vi "Buffer Classes Test.vi"() -> ()   [LabVIEW 2012]
uses:
  Engine/Classes/Waveforms/Buffer/Waveform Buffer/Waveform Buffer.lvclass
  Engine/Classes/Waveforms/Buffer/DBL Waveform Buffer/DBL Waveform Buffer.lvclass
  Engine/Classes/Waveforms/Buffer/Waveform Buffer/Buffer Data Type.ctl
  Engine/Classes/Waveforms/Buffer/Waveform Buffer/Time Range.ctl
  Engine/Classes/Waveforms/Buffer/Waveform Buffer/Data Point.ctl
  Engine/Classes/Waveforms/Buffer/Waveform Buffer/Wfm Segment.ctl
panel:
  out "DBL Buffer":refnum<class "DBL Waveform Buffer.lvclass">
  out "Cluster":T1={"Data"=[3000.0, 3001.0, 3002.0, 3003.0, 3004.0, 3005.0, 3006.0, 3007.0, 3008.0, 3009.0, 3010.0, 3011.0], "Segment Info"={"New Segment"=TRUE, "Wfm time"=timestamp(3449251614.0738325 s since 1904-01-01)}, "dt"=0.001}
  out "current time":timestamp=timestamp(3449251579.04933 s since 1904-01-01)
  out "Data":cluster{"Data":dbl[]}[](array[cluster])=[{"Data"=[3000.0, 3001.0, 3002.0, 3003.0, 3004.0, 3005.0, 3006.0, 3007.0, 3008.0, 3009.0, 3010.0, 3011.0]}]
  out "Wfm Segments":T2[](array[typedef])=[{"ID"=3, "Total samples"=12, "Start"={"Index"=0, "Wfm time"=timestamp(3449251614.0738325 s since 1904-01-01), "Receive time"=timestamp(3449251614.0738325 s since 1904-01-01)}, "Finish"={"Index"=11, "Wfm time"=timestamp(3449251614.0858326 s since 1904-01-01), "Receive time"=timestamp(3449251614.0858326 s since 1904-01-01)}}]
  in  "Read Wfms":bool
  in  "Time Range":T4={"Use Receive Time"=FALSE, "Start Time"=timestamp(3417715391.753 s since 1904-01-01), "Stop time"=timestamp(3480787391.753 s since 1904-01-01)}
  out "Waveform Buffer":refnum<class "Waveform Buffer.lvclass">
  in  "Send Wfm":bool
  in  "Wfm":T5={"New Segment"=TRUE, "dt"=0.001, "Wfm size"=12}
  in  "stop":bool
  in  "Buffer Duration":dbl=2.0
  in  "Buffer Data Type":T6
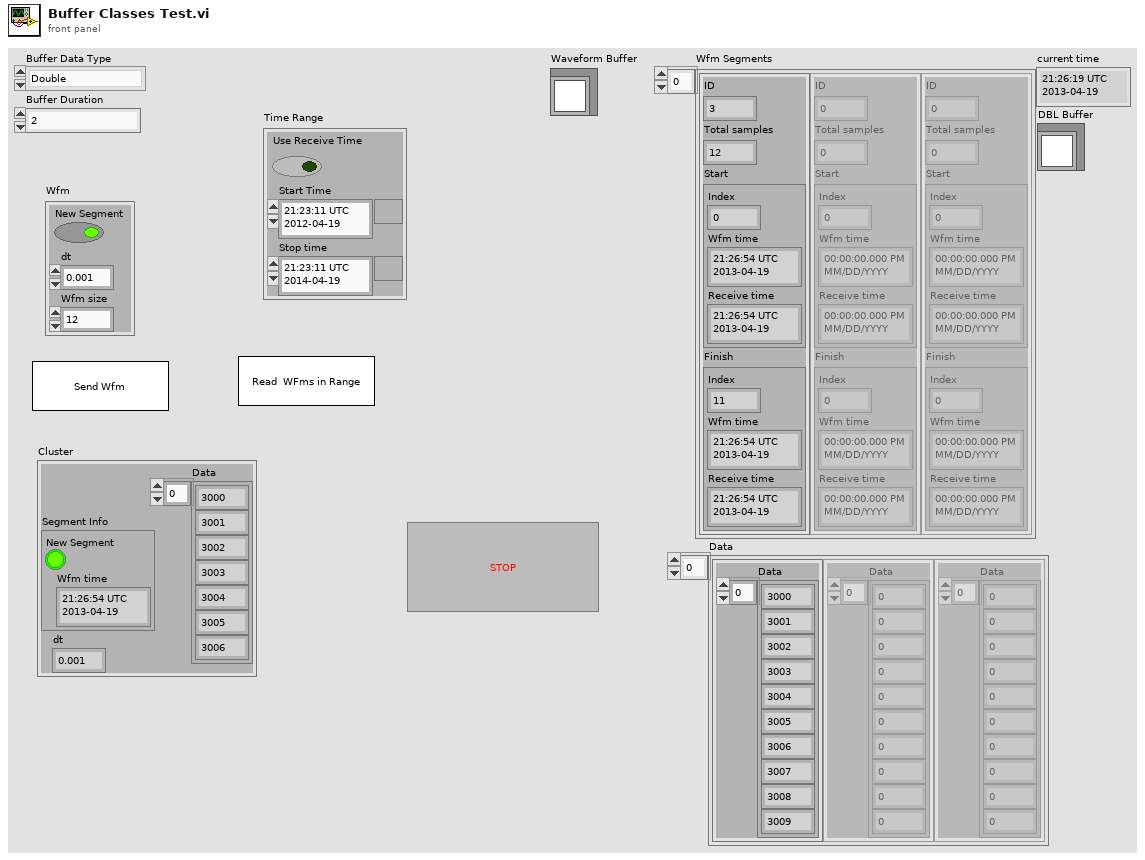
[diagram p1: front panel]
types:
  T1 = cluster{"Data":dbl[], "Segment Info":cluster{"New Segment":bool, "Wfm time":timestamp}, "dt":dbl}
  T2 = typedef "Waveform Data Logger Engine.lvlib/Waveform Buffer.lvclass/Wfm Segment.ctl" = cluster{"ID":u64, "Total samples":i32, "Start":T3, "Finish":T3}
  T3 = typedef "Waveform Data Logger Engine.lvlib/Waveform Buffer.lvclass/Data Point.ctl" = cluster{"Index":i32, "Wfm time":timestamp, "Receive time":timestamp}
  T4 = typedef "Waveform Data Logger Engine.lvlib/Waveform Buffer.lvclass/Time Range.ctl" = cluster{"Use Receive Time":bool, "Start Time":timestamp, "Stop time":timestamp}
  T5 = cluster{"New Segment":bool, "dt":dbl, "Wfm size":i32}
  T6 = typedef "Waveform Data Logger Engine.lvlib/Waveform Buffer.lvclass/Buffer Data Type.ctl" = enum16{"Double", "ComplexDouble"}
  T7 = cluster{"New Segment":bool, "Wfm time":timestamp, "Receive time":timestamp}
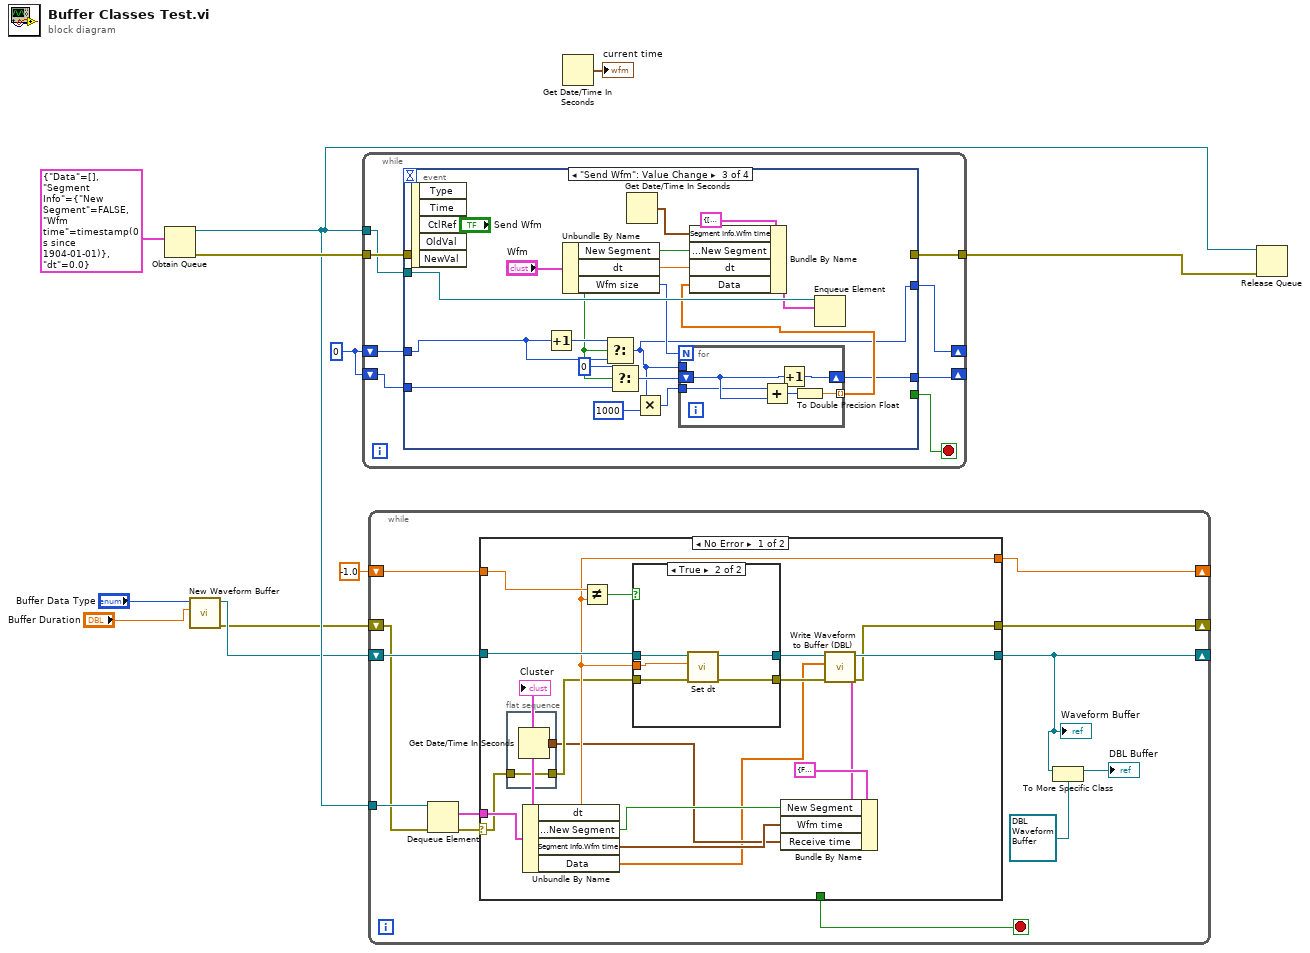
[diagram p0: block diagram]
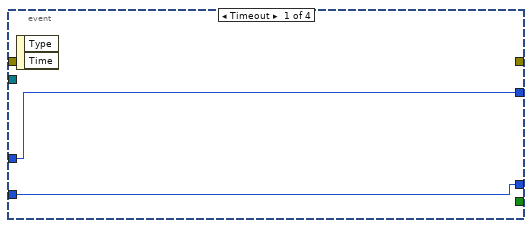
[diagram p2: hidden frame]
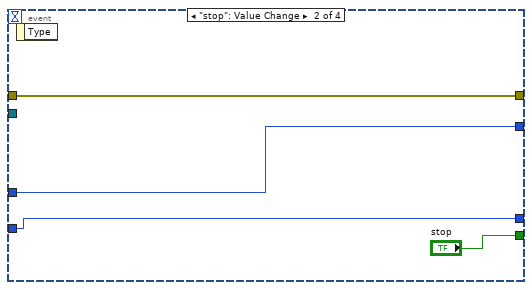
[diagram p3: hidden frame]
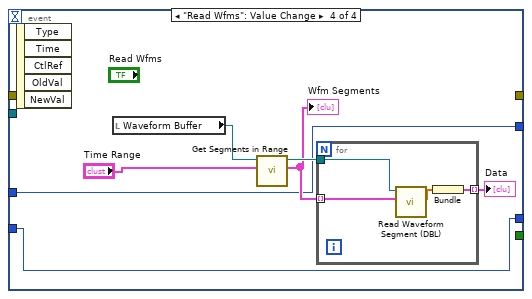
[diagram p4: hidden frame]
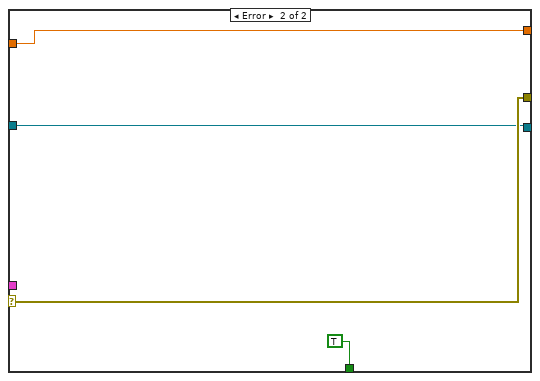
[diagram p6: hidden frame]
diagram:
  w5 = 0
  n1 = Obtain Queue(element data type=T1 {"Data"=[], "Segment Info"={"New Segment"=FALSE, "Wfm time"=timestamp(0 s since 1904-01-01)}, "dt"=0.0}) -> (queue out=w7:refnum<queue>, error out=w9:errorcluster)  [unwired: 4 in, 1 out]
  n2 = call "New Waveform Buffer.vi"("Buffer Duration"="Buffer Duration", "Buffer Data Type"="Buffer Data Type") -> ("error out"=w3:errorcluster, "Waveform Buffer out"=w4:refnum<class "Waveform Buffer.lvclass">)  [unwired: 8 in]
  n3 = while {
    tunnel: w7 -> [w14]
    tunnel: w9 -> [w17]
    tunnel: [w18] -> w8
    shift-right: [w16] -> _
    shift-left: w5 -> [w15]
    shift-right: [w12] -> _
    shift-left: w5 -> [w13]
    stop <- w19 stop-if-true
    n4 = event shown="[2] \"Send Wfm\": Value Change" {
      selector: _ -> [_ _ _ _]
      dyn-events: _ -> [_ _ _ _]
      timeout: _ -> [_ _ _ _]
      tunnel: [_ "stop" _ _] -> w19
      tunnel: [_ w24 _ _] -> w18
      tunnel: w17 -> [_ w24 _ _]
      tunnel: [w21 w23 w29 w50] -> w16
      tunnel: w15 -> [w21 w23 w41 w50]
      tunnel: w14 -> [_ _ w40 _]
      tunnel: w13 -> [w20 w22 w34 w49]
      tunnel: [w20 w22 w30 w49] -> w12
      event Timeout {
        n5 = event-data() -> ()  [unwired: 1 in, 2 out]
      }
      event "stop": Value Change {
        n6 = event-data() -> ()  [unwired: 1 in, 1 out]
      }
      event "Send Wfm": Value Change {
        n7 = event-data() -> ()  [unwired: 1 in, 5 out]
        n8 = Increment(x=w41) -> (x+1=w42:i32)
        n9 = Unbundle By Name("Wfm") -> ("New Segment"=w36:bool, "dt"=w38:dbl, "Wfm size"=w37:i32)
        n10 = Select(t=w42, s=w36, f=w41) -> (s? t:f=w29:i32)
        n11 = Select(t=0, s=w36, f=w34) -> (s? t:f=w33:i32)
        n12 = Get Date/Time In Seconds() -> (seconds since 1Jan1904=w26:timestamp)
        n13 = Multiply(x=w29, y=1000) -> (x*y=w27:i32)
        n14 = for {
          N: w37 -> [_]
          shift-right: [w46] -> w30
          shift-left: w33 -> [w45]
          tunnel: w29 -> [_]
          tunnel: [w47] -> w32 mode=indexing
          tunnel: w27 -> [w44]
          n15 = Add(x=w44, y=w45) -> (x+y=w48:i32)
          n16 = Increment(x=w45) -> (x+1=w46:i32)
          n17 = To Double Precision Float(number=w48) -> (double precision float=w47:dbl)
        }
        n18 = Bundle By Name(cluster=T1 {"Data"=[], "Segment Info"={"New Segment"=FALSE, "Wfm time"=timestamp(0 s since 1904-01-01)}, "dt"=0.0}, "Segment Info.Wfm time"=w26, "Segment Info.New Segment"=w36, "dt"=w38, "Data"=w32) -> (w31:T1)
        n19 = Enqueue Element(queue=w40, element=w31) -> ()  [unwired: 2 in, 3 out]
      }
      event "Read Wfms": Value Change {
        n20 = event-data() -> ()  [unwired: 1 in, 5 out]
        n21 = local read "Waveform Buffer"() -> (w55:refnum<class "Waveform Buffer.lvclass">)
        n22 = call "Get Segments in Range.vi"("Time Range"="Time Range", "Waveform Buffer in"=w55) -> ("Wfm Segments"=w52:T2[], "Waveform Buffer out"=w53:refnum<class "Waveform Buffer.lvclass">)  [unwired: 6 in, 2 out]
        "Wfm Segments" <- w52
        n23 = for {
          tunnel: w53 -> [w58]
          tunnel: w52 -> [w59] mode=indexing
          tunnel: [w56] -> w51 mode=indexing
          n24 = call "Read Waveform Segment (DBL).vi"("Wfm Segment"=w59, "Waveform Buffer in"=w58) -> ("Data"=w57:dbl[])  [unwired: 7 in, 2 out]
          n25 = Bundle("Data"=w57) -> (w56:cluster{"Data":dbl[]})  [unwired: 1 in]
        }
        "Data" <- w51
      }
    }
  }
  n26 = while {
    tunnel: w7 -> [w71]
    shift-right: [w65] -> _
    shift-left: -1.0 -> [w66]
    shift-right: [w62] -> _
    shift-left: w4 -> [w67]
    shift-right: [w63] -> _
    shift-left: w3 -> [w64]
    stop <- w69 stop-if-true
    n27 = Dequeue Element(queue=w71, error in (no error)=w64) -> (element=w68:T1, error out=w70:errorcluster)  [unwired: 1 in, 2 out]
    n28 = case shown="No Error" w70 {
      selector: w70 -> [w79 w99]
      tunnel: [_ TRUE] -> w69
      tunnel: w68 -> [w88 _]
      tunnel: w67 -> [w85 w98]
      tunnel: w66 -> [w87 w100]
      tunnel: [w84 w100] -> w65
      tunnel: [w81 w98] -> w62
      tunnel: [w80 w99] -> w63
      frame No Error {
        n29 = flat-sequence {
          tunnel: w79 -> [w90]
          tunnel: [w90] -> w78
          tunnel: [w89] -> w74
          frame #0 {
            n30 = Get Date/Time In Seconds() -> (seconds since 1Jan1904=w89:timestamp)
          }
        }
        n31 = Unbundle By Name(w88) -> ("dt"=w84:dbl, "Segment Info.New Segment"=w76:bool, "Segment Info.Wfm time"=w75:timestamp, "Data"=w72:dbl[])
        n32 = Not Equal?(x=w87, y=w84) -> (x != y?=w86:bool)
        n33 = case shown="True" w86 {
          tunnel: w85 -> [w91 w97]
          tunnel: w78 -> [w92 w96]
          tunnel: w84 -> [_ w95]
          tunnel: [w91 w94] -> w83
          tunnel: [w92 w93] -> w82
          frame False {
          }
          frame True {
            n34 = call "Set dt.vi"("error in (no error)"=w96, "dt"=w95, "Waveform Buffer in"=w97) -> ("error out"=w93:errorcluster, "Waveform Buffer out"=w94:refnum<class "Waveform Buffer.lvclass">)  [unwired: 7 in]
          }
        }
        n35 = Bundle By Name(cluster=T7 {"New Segment"=FALSE, "Wfm time"=timestamp(0 s since 1904-01-01), "Receive time"=timestamp(0 s since 1904-01-01)} ("Segment Info"), "New Segment"=w76, "Wfm time"=w75, "Receive time"=w74) -> (w73:T7)
        n36 = call "Write Waveform to Buffer (DBL).vi"("error in (no error)"=w82, "Waveform Info"=w73, "Data"=w72, "Waveform Buffer in"=w83) -> ("error out"=w80:errorcluster, "Waveform Buffer out"=w81:refnum<class "Waveform Buffer.lvclass">)  [unwired: 6 in]
        "Cluster" <- w88
      }
      frame Error {
      }
    }
    "Waveform Buffer" <- w62
    n37 = To More Specific Class(target class=refnum<class "DBL Waveform Buffer.lvclass"> refnum ("Waveform Data Logger Engine.lvlib:DBL Waveform Buffer.lvclass"), reference=w62) -> (specific class reference=→"DBL Buffer":refnum<class "DBL Waveform Buffer.lvclass">)  [unwired: 1 in, 1 out]
  }
  n38 = Get Date/Time In Seconds() -> (seconds since 1Jan1904=→"current time":timestamp)
  n39 = Release Queue(queue=w7, error in (no error)=w8) -> ()  [unwired: 1 in, 3 out]
